vi "SECoP_dataCreateDouble.vi"(6 "value":dbl, 8 "error in (no error)":errorcluster, 9 "maximum value":dbl=nan, 10 "minimum value":dbl=nan, 11 "DLL path (in)":T2) -> (0 "error out":errorcluster, 2 "SECoP_dataPtr (out)":T1 {"ptr64" format="%.0x"; "ptr32" format="%.0x"}, 3 "DLL path (out)":T2)   [LabVIEW 2023, in "SECoP.lvlib"]
doc: "Call <b>\"SECoP_dataCreateDouble.vi\"</b> to create a simple double (numeric) data type and set value. Free resources after use with <b>\"SECoP_dataDestroy.vi\"</b>.\n\n<b>DLL path</b> input and output of cluster from \"SECoP-Initialize.vi\"\n<b>minimum value</b> smallest allowed value or NaN\n<b>maximum value</b> greatest allowed value or NaN\n<b>value</b> new value\n<b>SECoP_dataPtr</b> created data"
uses:
  SECoP.lvlib
  SECoP-libraries.ctl
  SECoP-data.ctl
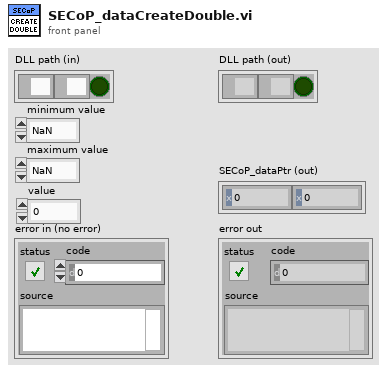
[diagram p1: front panel]
types:
  T1 = typedef "SECoP.lvlib/SECoP-data.ctl" = cluster{"ptr32":u32, "ptr64":u64}
  T2 = typedef "SECoP.lvlib/SECoP-libraries.ctl" = cluster{"serverDLL":path, "variantDLL":path, "cleanup_mode":bool}
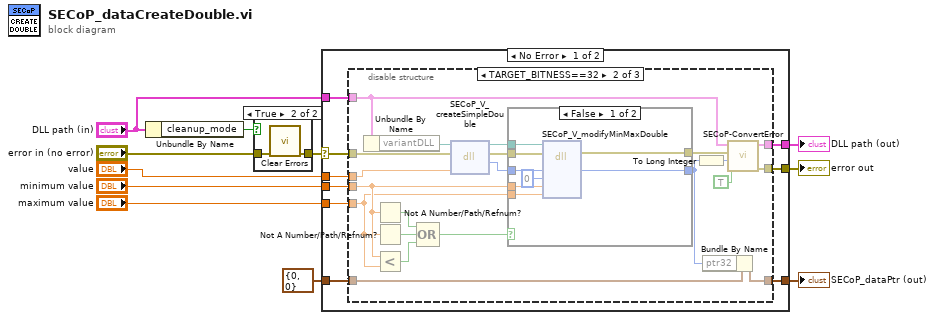
[diagram p0: block diagram]
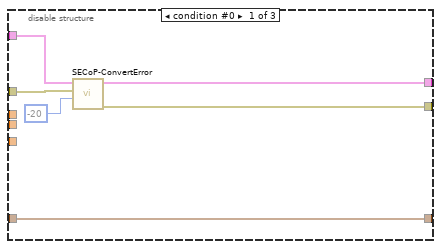
[diagram p3: hidden frame]
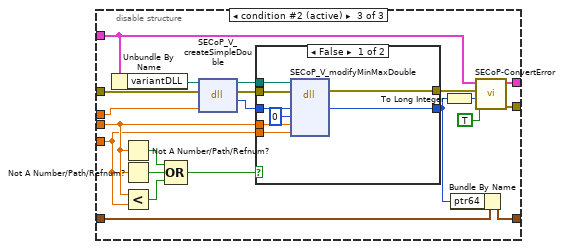
[diagram p5: hidden frame]
diagram:
  n1 = Unbundle By Name("DLL path (in)") -> ("cleanup_mode"=w9:bool)
  n2 = case shown="True" w9 {
    tunnel: "error in (no error)" -> [w12 w14]
    tunnel: [w12 w13] -> w7
    frame False {
    }
    frame True {
      n3 = call <vilib>:"Clear Errors.vi"("error in (no error)"=w14) -> ("error out"=w13:errorcluster)  [unwired: 5 in, 1 out]
    }
  }
  n4 = case shown="No Error" w7 {
    selector: w7 -> [w23 w93]
    tunnel: "DLL path (in)" -> [w22 w94]
    tunnel: [w20 w94] -> w11
    tunnel: [w21 w93] -> w10
    tunnel: [w18 w92] -> w6
    tunnel: T1 {"ptr32"=0, "ptr64"=0} ("SECoP_dataPtr (out)") -> [w19 w92]
    tunnel: "minimum value" -> [w17 _]
    tunnel: "maximum value" -> [w16 _]
    tunnel: "value" -> [w15 _]
    frame No Error {
      n5 = disable-structure shown="TARGET_BITNESS==32" {
        disable-tunnel: w23 -> [w29 w50 w81]
        disable-tunnel: w22 -> [w28 w30 w61]
        disable-tunnel: [w26 w47 w78] -> w21
        disable-tunnel: [w27 w46 w77] -> w20
        disable-tunnel: w19 -> [w24 w48 w79]
        disable-tunnel: [w24 w49 w80] -> w18
        disable-tunnel: w17 -> [_ w34 w65]
        disable-tunnel: w16 -> [_ w33 w64]
        disable-tunnel: w15 -> [_ w32 w63]
        frame condition #0 {
          n6 = call "SECoP-ConvertError.vi"("return code"=-20, "error in (no error)"=w29, "DLL path (in)"=w28) -> ("error out"=w26:errorcluster, "DLL path (out)"=w27:T2)  [unwired: 7 in]
        }
        frame condition #1 {
          n7 = Unbundle By Name(w30) -> ("variantDLL"=w31:path)
          n8 = Not A Number/Path/Refnum?(number/path/refnum=w34) -> (NaN/Path/Refnum?=w38:bool)
          n9 = Not A Number/Path/Refnum?(number/path/refnum=w33) -> (NaN/Path/Refnum?=w37:bool)
          n10 = Less?(x=w34, y=w33) -> (x < y?=w36:bool)
          n11 = Compound Arithmetic op=OR(w38, w37, w36) -> (w35:bool)
          n12 = dll-call lib="Z:/Praktische_Aufgaben/SECoP-LabVIEW2015/32bit/SECoP32.dll" fn="SECoP_V_createSimpleDouble"(path in=w31, error in=w50, "dValue"=w32) -> (path out=w43:path, error out=w42:errorcluster, "return type"=w40:u32)  [unwired: 2 in]
          n13 = case shown="False" w35 {
            tunnel: w43 -> [w58 _]
            tunnel: w42 -> [w57 w60]
            tunnel: [w56 w60] -> w41
            tunnel: w40 -> [w55 w59]
            tunnel: [w54 w59] -> w39
            tunnel: w34 -> [w52 _]
            tunnel: w33 -> [w51 _]
            frame False {
              n14 = dll-call lib="Z:/Praktische_Aufgaben/SECoP-LabVIEW2015/32bit/SECoP32.dll" fn="SECoP_V_modifyMinMaxDouble"(path in=w58, error in=w57, "pData"=w55, "uPosition"=u32 0, "dMinimum"=w52, "dMaximum"=w51) -> (error out=w56:errorcluster, "pData"=w54:u32)  [unwired: 5 in, 1 out]
            }
            frame True {
            }
          }
          n15 = To Long Integer(number=w39) -> (32bit integer=w44:i32)
          n16 = Bundle By Name(cluster=w48, "ptr32"=w39) -> (w49:T1)
          n17 = call "SECoP-ConvertError.vi"("return is boolean"=TRUE, "return code"=w44, "error in (no error)"=w41, "DLL path (in)"=w30) -> ("error out"=w47:errorcluster, "DLL path (out)"=w46:T2)  [unwired: 6 in]
        }
        frame condition #2 (active) {
          n18 = Unbundle By Name(w61) -> ("variantDLL"=w62:path)
          n19 = Not A Number/Path/Refnum?(number/path/refnum=w65) -> (NaN/Path/Refnum?=w69:bool)
          n20 = Not A Number/Path/Refnum?(number/path/refnum=w64) -> (NaN/Path/Refnum?=w68:bool)
          n21 = Less?(x=w65, y=w64) -> (x < y?=w67:bool)
          n22 = Compound Arithmetic op=OR(w69, w68, w67) -> (w66:bool)
          n23 = dll-call lib="Z:/Praktische_Aufgaben/SECoP-LabVIEW2015/32bit/SECoP32.dll" fn="SECoP_V_createSimpleDouble"(path in=w62, error in=w81, "dValue"=w63) -> (path out=w74:path, error out=w73:errorcluster, "return type"=w71:u64)  [unwired: 2 in]
          n24 = case shown="False" w66 {
            tunnel: w74 -> [w89 _]
            tunnel: w73 -> [w88 w91]
            tunnel: [w87 w91] -> w72
            tunnel: w71 -> [w86 w90]
            tunnel: [w85 w90] -> w70
            tunnel: w65 -> [w83 _]
            tunnel: w64 -> [w82 _]
            frame False {
              n25 = dll-call lib="Z:/Praktische_Aufgaben/SECoP-LabVIEW2015/32bit/SECoP32.dll" fn="SECoP_V_modifyMinMaxDouble"(path in=w89, error in=w88, "pData"=w86, "uPosition"=u32 0, "dMinimum"=w83, "dMaximum"=w82) -> (error out=w87:errorcluster, "pData"=w85:u64)  [unwired: 5 in, 1 out]
            }
            frame True {
            }
          }
          n26 = To Long Integer(number=w70) -> (32bit integer=w75:i32)
          n27 = Bundle By Name(cluster=w79, "ptr64"=w70) -> (w80:T1)
          n28 = call "SECoP-ConvertError.vi"("return is boolean"=TRUE, "return code"=w75, "error in (no error)"=w72, "DLL path (in)"=w61) -> ("error out"=w78:errorcluster, "DLL path (out)"=w77:T2)  [unwired: 6 in]
        }
      }
    }
    frame Error {
    }
  }
  "DLL path (out)" <- w11
  "error out" <- w10
  "SECoP_dataPtr (out)" <- w6
